vi "rampRatesToSetpoints.vi"(9 "Room Temperature":dbl=30.0, 10 "Ramp Rates":cluster{"Duration (m)":dbl, "Rate (C/m)":dbl}[](array[cluster])) -> (2 "Setpoint Profile":cluster{"Time (s)":dbl, "Setpoint (C)":dbl}[](array[cluster]))   [LabVIEW 2018]
panel:
  # "Converts Ramp Rates to Setpoint Profile for use with Default Labview Controller\nTime = f(t0, dt) = t0 + dt *** Notice conversion from minutes to seconds ***\nSetpoint = g(y0, dy/dt, dt) = y0 + (dy/dt)*dt"
  # "***Room Temperature Assumed 30 C if left blank***"
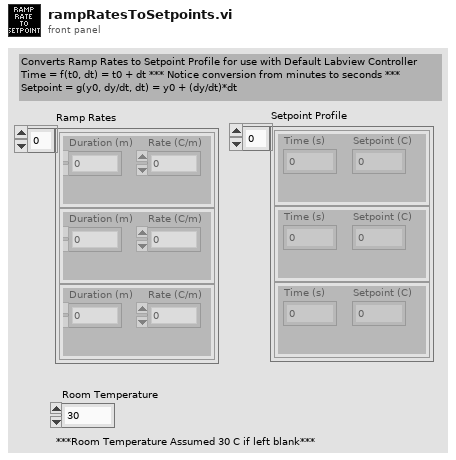
[diagram p1: front panel]
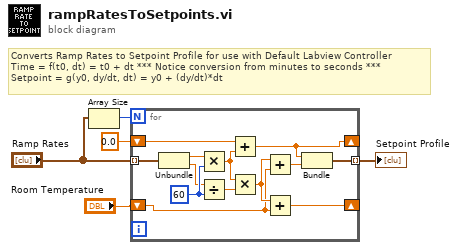
[diagram p0: block diagram]
diagram:
  # "Converts Ramp Rates to Setpoint Profile for use with Default Labview Controller\nTime = f(t0, dt) = t0 + dt *** Notice conversion from minutes to seconds ***\nSetpoint = g(y0, dy/dt, dt) = y0 + (dy/dt)*dt"
  n1 = Array Size(array="Ramp Rates") -> (size(s)=w3:i32)
  n2 = for {
    N: w3 -> [_]
    tunnel: "Ramp Rates" -> [w18] mode=indexing
    shift-right: [w10] -> _
    shift-left: 0.0 -> [w14]
    shift-right: [w9] -> _
    shift-left: "Room Temperature" -> [w6]
    tunnel: [w13] -> w4 mode=indexing
    w16 = 60
    n3 = Unbundle(w18) -> ("Duration (m)"=w17:dbl, "Rate (C/m)"=w15:dbl)
    n4 = Multiply(x=w17, y=w16) -> (x*y=w12:dbl)
    n5 = Divide(x=w15, y=w16) -> (x/y=w11:dbl)
    n6 = Add(x=w14, y=w12) -> (x+y=w10:dbl)
    n7 = Multiply(x=w12, y=w11) -> (x*y=w8:dbl)
    n8 = Add(x=w8, y=w6) -> (x+y=w7:dbl)
    n9 = Add(x=w8, y=w6) -> (x+y=w9:dbl)
    n10 = Bundle(w10, w7) -> (w13:cluster{dbl, dbl})  [unwired: 1 in]
  }
  "Setpoint Profile" <- w4
